vi "FilterAndConvertToString.vi"(8 "Max noise amplitude":dbl, 9 "Y":dbl[][](array[numeric]), 10 "dt":dbl, 11 "t":dbl) -> (3 "String":string)   [LabVIEW 2009]
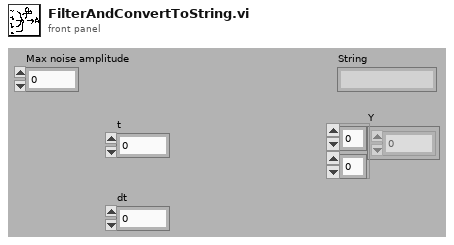
[diagram p1: front panel]
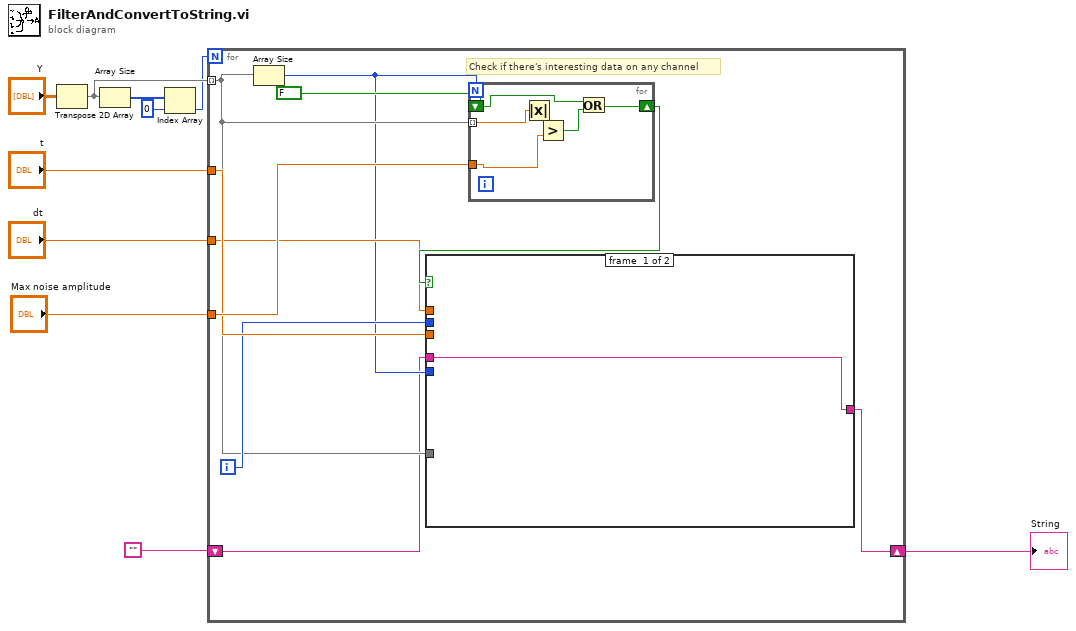
[diagram p0: block diagram]
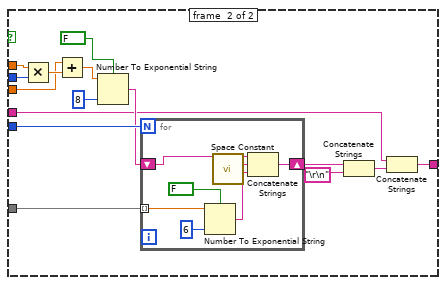
[diagram p2: hidden frame]
diagram:
  n1 = Transpose 2D Array(2D array="Y") -> (transposed array=w9:dbl[][])
  n2 = Array Size(array=w9) -> (size(s)=w8:i32[])
  n3 = Index Array(array=w8, index=0) -> (element=w7:i32)
  n4 = for {
    N: w7 -> [_]
    tunnel: w9 -> [w14] mode=indexing
    tunnel: "t" -> [w17]
    tunnel: "dt" -> [w16]
    tunnel: "Max noise amplitude" -> [w20]
    shift-right: [w11] -> w1
    shift-left: "" -> [w12]
    i -> [w15]
    # "Check if there's interesting data on any channel"
    n5 = Array Size(array=w14) -> (size(s)=w13:i32)
    n6 = for {
      N: w13 -> [_]
      tunnel: w14 -> [w44] mode=indexing
      tunnel: w20 -> [w48]
      shift-right: [w47] -> w18
      shift-left: FALSE -> [w46]
      n7 = Absolute Value(x=w44) -> (abs(x)=w49:dbl)
      n8 = Greater?(x=w49, y=w48) -> (0:w45:bool)
      n9 = Or(x=w46, y=w45) -> (x .or. y?=w47:bool)
    }
    n10 = case shown="True" w18 {
      tunnel: w17 -> [_ w35]
      tunnel: w16 -> [_ w34]
      tunnel: w15 -> [_ w33]
      tunnel: w14 -> [_ w32]
      tunnel: w13 -> [_ w31]
      tunnel: w12 -> [w21 w24]
      tunnel: [w21 w22] -> w11
      frame #0 {
      }
      frame #1 {
        n11 = Multiply(x=w34, y=w33) -> (x*y=w36:dbl)
        n12 = Add(x=w35, y=w36) -> (x+y=w28:dbl)
        n13 = Number To Exponential String(number=w28, precision (6)=i16 8, 1:FALSE ("use system decimal point (T)")) -> (E-format string=w27:string)  [unwired: 1 in]
        n14 = for {
          N: w31 -> [_]
          tunnel: w32 -> [w41] mode=indexing
          shift-right: [w37] -> w26
          shift-left: w27 -> [w40]
          n15 = Number To Exponential String(number=w41, precision (6)=i16 6, 1:FALSE ("use system decimal point (T)")) -> (E-format string=w38:string)  [unwired: 1 in]
          n16 = call <vilib>:"Space Constant.vi"() -> ("String"=w39:string)
          n17 = Concatenate Strings(w40, w39, w38) -> (w37:string)
        }
        n18 = Concatenate Strings(w26, "\r\n") -> (w23:string)
        n19 = Concatenate Strings(w24, w23) -> (w22:string)
      }
    }
  }
  "String" <- w1
